vi "OAD.vi"(0 "System no.":i32=1 min=1 max=4 step=1, 2 "Channels to set":string[](array[string]), 3 "Driving voltage":dbl[](array[numeric]) format="%.6f", 4 "No.of digits":i16=4, 5 "error in":errorcluster) -> (14 "Controller error":bool, 19 "error out":errorcluster)   [LabVIEW 2020]
doc: "Sets driving voltage amplitude of open-loop analog driving for given PiezoWalk channels. No. of digits is the number of digits after the decimal point in the voltage value(s) that will be sent. Hidden error is TRUE if selected system reports error code which is not 0.\n\nE-861: Servo must be disabled for the commanded axis prior to using this command (open-loop operation). In open-loop operation, an RNP command must be sent each time the motion mode is to be changed from stepping motion (OSM command) to analog motion (OAD command) and vice versa. RNP brings the drive to a full-holding-force, zero-drive-voltage Relaxed state.\nThe first OAD sent for a NEXACT® linear drive which is in the Relaxed state prepares the drive for analog motion (brings it to the Analog state) before the actual motion is done. Once the drive is in the Analog state, each subsequent OAD motion will be executed immediately.\nThe first OAD after a change of motion mode and the RNP procedure can take up to four times the slewrate value (parameter ID 0x7000002; can be changed with SPA and SEP).\nAfter open-loop analog motion was done with OAD, an RNP command must be sent before the servo can be switched on with SVO for closed-loop operation.\nMotion commands like OAD are not allowed when a joystick is active on the axis."
panel:
  # "Sets driving voltage amplitude of open-loop analog driving for \ngiven PiezoWalk channels."
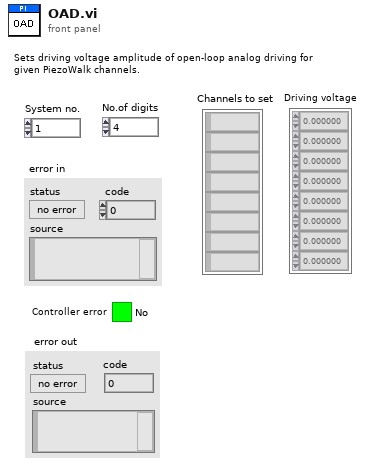
[diagram p1: front panel]
types:
  T1 = enum16{"Disable error check", "Force error check", "Use global settings"}
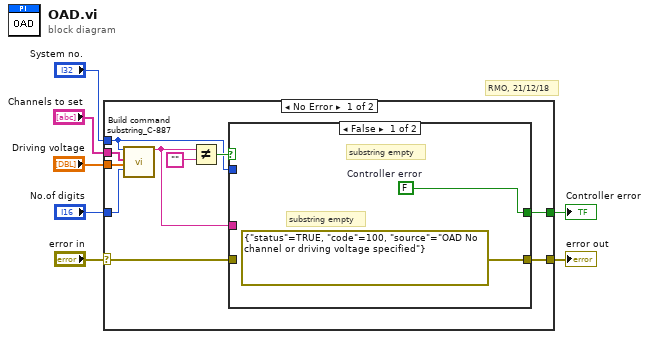
[diagram p0: block diagram]
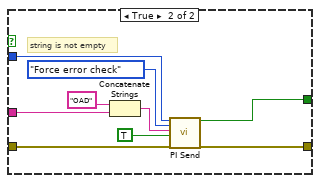
[diagram p2: hidden frame]
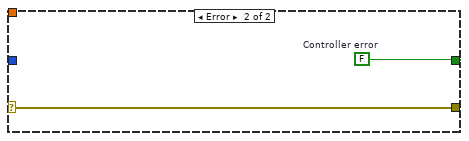
[diagram p3: hidden frame]
diagram:
  # "RMO, 21/12/18"
  n1 = case shown="No Error" "error in" {
    selector: "error in" -> [w8 w30]
    tunnel: [w17 w30] -> w7
    tunnel: "Driving voltage" -> [w14 _]
    tunnel: "No.of digits" -> [w13 _]
    tunnel: "System no." -> [w10 _]
    tunnel: "Channels to set" -> [w12 _]
    tunnel: [w9 w29] -> w2
    frame No Error {
      n2 = call "Build command substring_C-887.vi"("System no."=w10, "Affected axes"=w12, "Parameters"=w14, "No. of digits"=w13) -> ("Command substring"=w15:string)  [unwired: 3 in, 12 out]
      n3 = Not Equal?(x=w15, y="") -> (x != y?=w11:bool)
      n4 = case shown="False" w11 {
        tunnel: w15 -> [_ w27]
        tunnel: [errorcluster {"status"=TRUE, "code"=100, "source"="OAD No channel or driving voltage specified"} ("error out") w21] -> w17
        tunnel: w8 -> [_ w24]
        tunnel: w10 -> [_ w23]
        tunnel: [w18 w22] -> w9
        frame False {
          w18 = FALSE  # Controller error
          # "substring empty"
          # "substring empty"
        }
        frame True {
          # "string is not empty"
          n5 = Concatenate Strings("OAD", w27) -> (w25:string)
          n6 = call "PI Send.vi"("System no."=w23, "Error check settings"=T1."Force error check", "String to send"=w25, "Attach termination char.?"=TRUE ("Attach Linefeed?"), "error in"=w24) -> ("Controller error"=w22:bool, "error out"=w21:errorcluster)  [unwired: 1 in, 12 out]
        }
      }
    }
    frame Error {
      w29 = FALSE  # Controller error
    }
  }
  "error out" <- w7
  "Controller error" <- w2
